vi "LED Brightess Control.vi"() -> ()   [LabVIEW 2022 SP3]
panel:
  out "Boolean":bool
  in  "Numeric 2":dbl
  in  "VISA resource name 2":refnum<visa-resource-name>
  out "Connected 2":bool
  in  "Connect":bool
  in  "Numeric":dbl
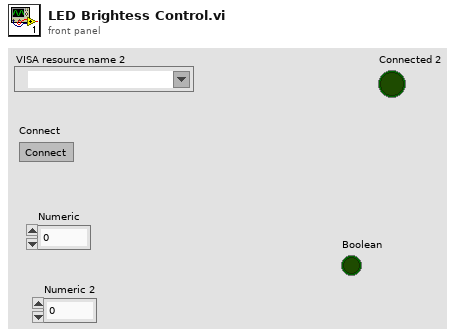
[diagram p1: front panel]
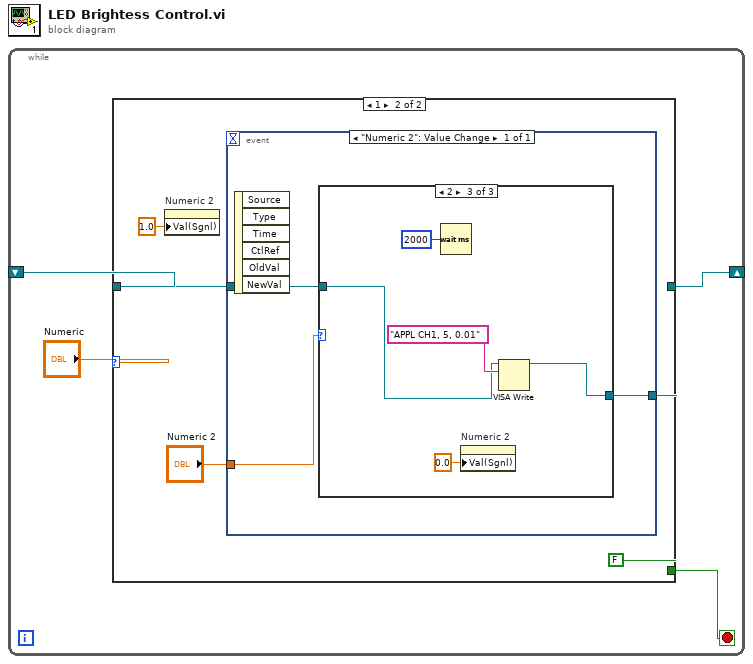
[diagram p0: block diagram]
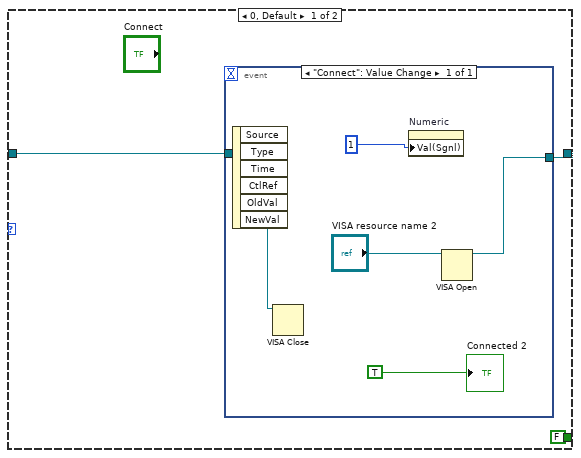
[diagram p2: hidden frame]
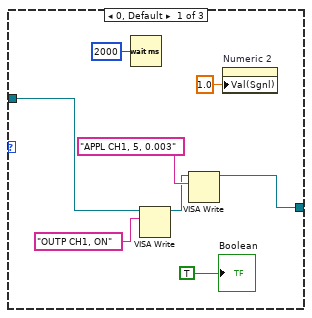
[diagram p3: hidden frame]
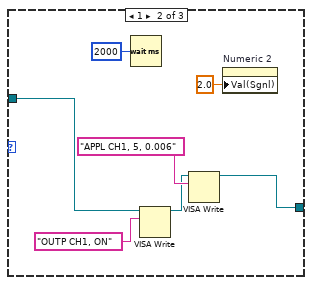
[diagram p4: hidden frame]
diagram:
  n1 = while {
    shift-right: [w3] -> _
    shift-left: _ -> [w4]
    stop <- w1 stop-if-true
    n2 = case shown="1" "Numeric" {
      tunnel: w4 -> [w7 w17]
      tunnel: [w6 w16] -> w3
      tunnel: [FALSE FALSE] -> w1
      frame 0, Default {
        n3 = event shown="[0] \"Connect\": Value Change" {
          selector: _ -> [_]
          dyn-events: _ -> [_]
          timeout: _ -> [_]
          tunnel: [w11] -> w6
          tunnel: w7 -> [w9]
          event "Connect": Value Change {
            n4 = event-data() -> ()  [unwired: 1 in, 6 out]
            n5 = VISA Close(VISA resource name=w9) -> ()  [unwired: 1 in, 1 out]
            n6 = property on="Numeric" class="DigNum (strict)"("Val(Sgnl)"=1) -> ()  [unwired: 2 in, 2 out]
            n7 = VISA Open(VISA resource name="VISA resource name 2") -> (VISA resource name=w11:refnum<visa-resource-name>)  [unwired: 4 in, 1 out]
            "Connected 2" <- TRUE
          }
        }
      }
      frame 1 {
        n8 = property on="Numeric 2" class="DigNum (strict)"("Val(Sgnl)"=1.0 ("Value (Signaling)")) -> ()  [unwired: 2 in, 2 out]
        n9 = event shown="[0] \"Numeric 2\": Value Change" {
          selector: _ -> [_]
          dyn-events: _ -> [_]
          timeout: _ -> [_]
          tunnel: w17 -> [w20]
          tunnel: [w19] -> w16
          tunnel: "Numeric 2" -> [w18]
          event "Numeric 2": Value Change {
            n10 = event-data() -> ()  [unwired: 1 in, 6 out]
            n11 = case shown="2" w18 {
              tunnel: w20 -> [w24 w31 w37]
              tunnel: [w23 w30 w38] -> w19
              frame 0, Default {
                n12 = Wait (ms)(milliseconds to wait=u32 2000) -> ()  [unwired: 1 out]
                n13 = VISA Write(VISA resource name=w24, write buffer="OUTP CH1, ON") -> (VISA resource name out=w26:refnum<visa-resource-name>)  [unwired: 1 in, 2 out]
                n14 = VISA Write(VISA resource name=w26, write buffer="APPL CH1, 5, 0.003") -> (VISA resource name out=w23:refnum<visa-resource-name>)  [unwired: 1 in, 2 out]
                n15 = property on="Numeric 2" class="DigNum (strict)"("Val(Sgnl)"=1.0 ("Value (Signaling)")) -> ()  [unwired: 2 in, 2 out]
                "Boolean" <- TRUE
              }
              frame 1 {
                n16 = Wait (ms)(milliseconds to wait=u32 2000) -> ()  [unwired: 1 out]
                n17 = VISA Write(VISA resource name=w31, write buffer="OUTP CH1, ON") -> (VISA resource name out=w33:refnum<visa-resource-name>)  [unwired: 1 in, 2 out]
                n18 = VISA Write(VISA resource name=w33, write buffer="APPL CH1, 5, 0.006") -> (VISA resource name out=w30:refnum<visa-resource-name>)  [unwired: 1 in, 2 out]
                n19 = property on="Numeric 2" class="DigNum (strict)"("Val(Sgnl)"=2.0 ("Value (Signaling)")) -> ()  [unwired: 2 in, 2 out]
              }
              frame 2 {
                n20 = Wait (ms)(milliseconds to wait=u32 2000) -> ()  [unwired: 1 out]
                n21 = property on="Numeric 2" class="DigNum (strict)"("Val(Sgnl)"=0.0 ("Value (Signaling)")) -> ()  [unwired: 2 in, 2 out]
                n22 = VISA Write(VISA resource name=w37, write buffer="APPL CH1, 5, 0.01") -> (VISA resource name out=w38:refnum<visa-resource-name>)  [unwired: 1 in, 2 out]
              }
            }
          }
        }
      }
    }
  }
